vi "URI Encode.vi"(8 "error in (no error)":errorcluster, 10 "URL":string) -> (0 "error out":errorcluster, 2 "URI out":string)   [LabVIEW 2012]
doc: "This VI should encode any special characters according to: http://en.wikipedia.org/wiki/Percent-encoding\n\nCurrently it just replaces all spaces (\" \") with plus signs (\"+\")."
uses:
  <vilib>/wsapi/NI_WebServices.lvlib
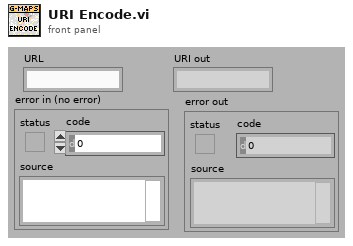
[diagram p1: front panel]
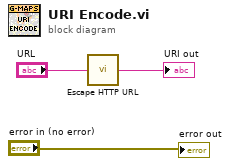
[diagram p0: block diagram]
diagram:
  n1 = call <vilib>:"Escape HTTP URL.vi"("unescaped string in"="URL") -> ("escaped string out"=→"URI out":string)
  "error out" <- "error in (no error)"
